vi "Day 14-Initialize Letter Count.vi"(11 "Initial Letters":u8[](array[numeric])) -> (3 "Count Array":u64[](array[numeric]))   [LabVIEW 2021]
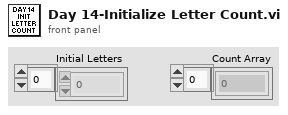
[diagram p1: front panel]
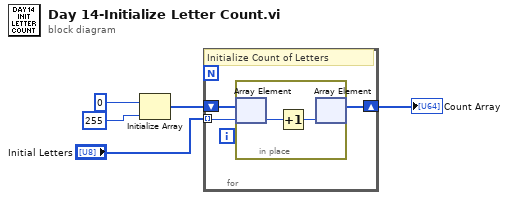
[diagram p0: block diagram]
diagram:
  n1 = Initialize Array(u64 0 ("element"), 255 ("dimension size")) -> (w5:u64[])
  n2 = for {
    shift-right: [w6] -> w1
    shift-left: w5 -> [w8]
    tunnel: "Initial Letters" -> [w7] mode=indexing
    # "Initialize Count of Letters"
    n3 = in-place {
      n4 = in-place-array #1(w8, w7) -> (w10:u64)
      n5 = Increment(x=w10) -> (x+1=w9:u64)
      n6 = in-place-array #1(w9) -> (w6:u64[])  [unwired: 1 out]
    }
  }
  "Count Array" <- w1
